vi "Configure Current Limit.vi"(8 "error in (no error)":errorcluster, 10 "Current Limit":dbl, 11 "Power Supply in":refnum<class "Power Supply.lvclass">) -> (0 "error out":errorcluster, 3 "Power Supply out":refnum<class "Power Supply.lvclass">)   [LabVIEW 2020, in "Power Supply.lvclass"]
uses:
  Power Supply.lvclass
  Power Supply.lvclass/Power Supply.ctl
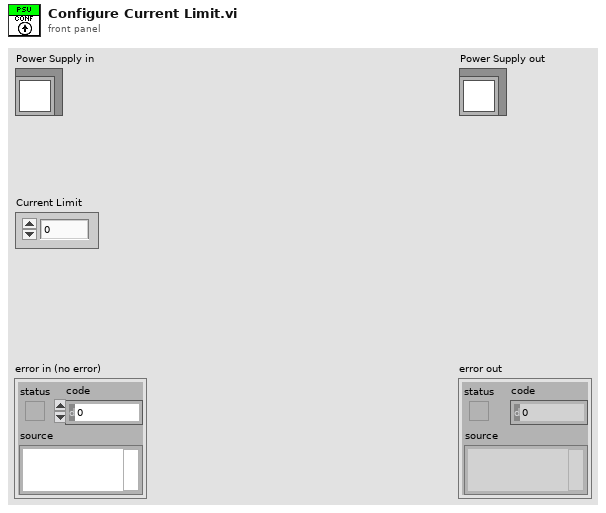
[diagram p1: front panel]
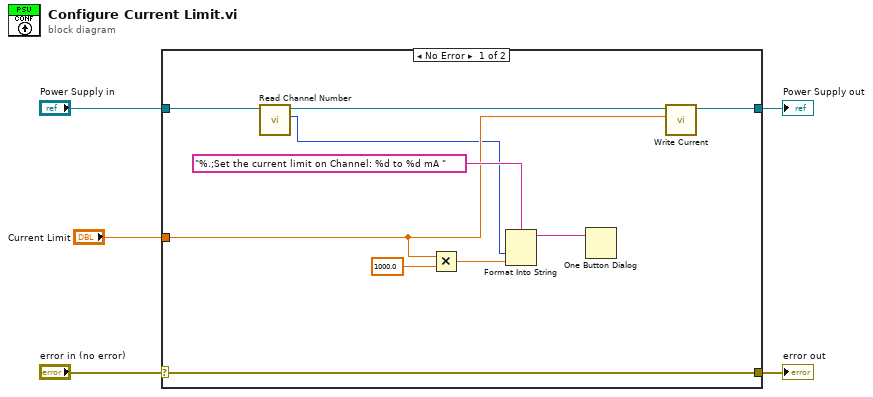
[diagram p0: block diagram]
diagram:
  n1 = case shown="No Error" "error in (no error)" {
    selector: "error in (no error)" -> [w15 w17]
    tunnel: [w15 w17] -> w4
    tunnel: [w10 w16] -> w2
    tunnel: "Power Supply in" -> [w8 w16]
    tunnel: "Current Limit" -> [w9 _]
    frame No Error {
      n2 = call "Read Channel Number.vi"("Power Supply in"=w8) -> ("Channel Number"=w6:u8, "Power Supply out"=w7:refnum<class "Power Supply.lvclass">)  [unwired: 9 in]
      n3 = Multiply(x=w9, y=1000.0) -> (x*y=w13:dbl)
      n4 = Format Into String(format string="%.;Set the current limit on Channel: %d to %d mA ", w6, w13) -> (resulting string=w11:string)  [unwired: 2 in, 1 out]
      n5 = One Button Dialog(message=w11) -> ()  [unwired: 1 in, 1 out]
      n6 = call "Write Current.vi"("Current"=w9, "Power Supply in"=w7) -> ("Power Supply out"=w10:refnum<class "Power Supply.lvclass">)  [unwired: 9 in]
    }
    frame Error {
    }
  }
  "error out" <- w4
  "Power Supply out" <- w2
